vi "SP Format Fundamental Value for Display (array).vi"(4 "dF, MHz":dbl, 6 "Formatted Data? (F)":bool, 8 "Display Format":T1, 9 "Fundamental Values":dbl[](array[numeric])) -> (1 "Formatted Values":dbl[](array[numeric]))   [LabVIEW 2011]
uses:
  TypeDefs/SP Format.ctl
  <vilib>/Analysis/NI_AALPro.lvlib
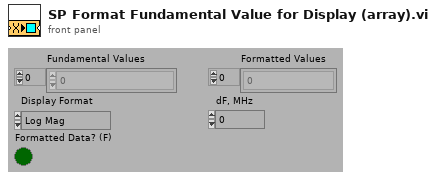
[diagram p1: front panel]
types:
  T1 = typedef "SP Format.ctl" = enum16{"Log Mag", "Lin Mag", "SWR", "Phase", "Expanded Phase", "Delay", "Insertion Loss", "Isolation", "Return Loss"}
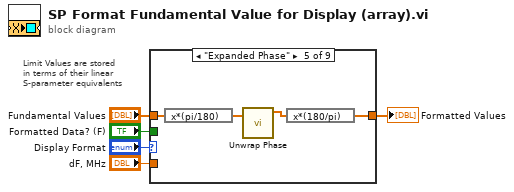
[diagram p0: block diagram]
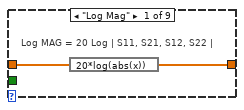
[diagram p2: hidden frame]
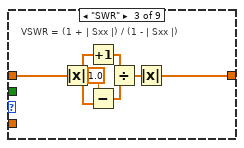
[diagram p4: hidden frame]
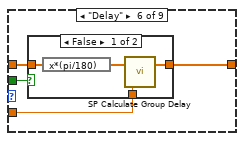
[diagram p6: hidden frame]
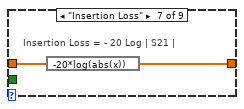
[diagram p8: hidden frame]
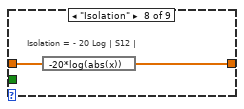
[diagram p9: hidden frame]
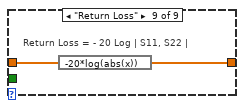
[diagram p10: hidden frame]
diagram:
  # "Limit Values are stored\nin terms of their linear\nS-parameter equivalents"
  n1 = case shown="\"Expanded Phase\"" "Display Format" {
    tunnel: [w7 w8 w9 w16 w17 w23 w31 w33 w35] -> w3
    tunnel: "Fundamental Values" -> [w6 w8 w11 w16 w20 w24 w30 w32 w34]
    tunnel: "dF, MHz" -> [_ _ _ _ _ w22 _ _ _]
    tunnel: "Formatted Data? (F)" -> [_ _ _ _ _ w21 _ _ _]
    frame "Log Mag" {
      # "Log MAG = 20 Log | S11, S21, S12, S22 |"
      n2 = expression code="20*log(abs(x))"(w6) -> (w7:dbl[])
    }
    frame "Lin Mag" {
    }
    frame "SWR" {
      # "VSWR = (1 + | Sxx |) / (1 - | Sxx |)"
      n3 = Absolute Value(x=w11) -> (abs(x)=w10:dbl[])
      n4 = Increment(x=w10) -> (x+1=w15:dbl[])
      n5 = Subtract(x=1.0, y=w10) -> (x-y=w13:dbl[])
      n6 = Divide(x=w15, y=w13) -> (x/y=w12:dbl[])
      n7 = Absolute Value(x=w12) -> (abs(x)=w9:dbl[])
    }
    frame "Phase" {
    }
    frame "Expanded Phase" {
      n8 = expression code="x*(pi/180)"(w20) -> (w19:dbl[])
      n9 = call <vilib>:"Unwrap Phase.vi"("Phase"=w19) -> ("Unwrapped Phase"=w18:dbl[])  [unwired: 1 in, 9 out]
      n10 = expression code="x*(180/pi)"(w18) -> (w17:dbl[])
    }
    frame "Delay" {
      n11 = case shown="False" w21 {
        tunnel: w24 -> [w27 w29]
        tunnel: [w26 w29] -> w23
        tunnel: w22 -> [w25 _]
        frame False {
          n12 = expression code="x*(pi/180)"(w27) -> (w28:dbl[])
          n13 = call "SP Calculate Group Delay.vi"("dF, MHz"=w25, "Phase, radians"=w28) -> ("Group Delay, seconds"=w26:dbl[])  [unwired: 1 out]
        }
        frame True {
        }
      }
    }
    frame "Insertion Loss" {
      # "Insertion Loss = - 20 Log | S21 |"
      n14 = expression code="-20*log(abs(x))"(w30) -> (w31:dbl[])
    }
    frame "Isolation" {
      # "Isolation = - 20 Log | S12 |"
      n15 = expression code="-20*log(abs(x))"(w32) -> (w33:dbl[])
    }
    frame "Return Loss" {
      # "Return Loss = - 20 Log | S11, S22 |"
      n16 = expression code="-20*log(abs(x))"(w34) -> (w35:dbl[])
    }
  }
  "Formatted Values" <- w3
